vi "ReadLampState.vi"(8 "error in (no error)":errorcluster, 11 "RoomLight in":refnum<class "RoomLight.lvclass">) -> (0 "error out":errorcluster, 2 "LampState":bool, 3 "RoomLight out":refnum<class "RoomLight.lvclass">)   [LabVIEW 2013, in "RoomLight.lvclass"]
uses:
  RoomLight.lvclass
  RoomLight.lvclass/RoomLight.ctl
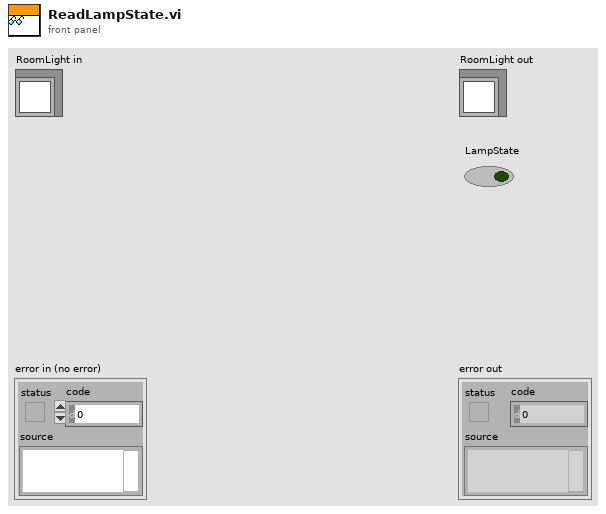
[diagram p1: front panel]
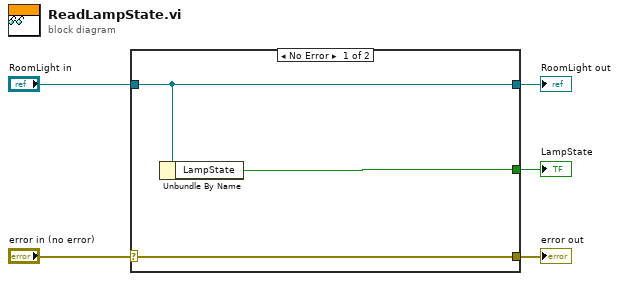
[diagram p0: block diagram]
diagram:
  n1 = case shown="No Error" "error in (no error)" {
    selector: "error in (no error)" -> [w8 w9]
    tunnel: [w8 w9] -> w4
    tunnel: [w7 w10] -> w2
    tunnel: "RoomLight in" -> [w7 w10]
    tunnel: [w6 _] -> w1
    frame No Error {
      n2 = Unbundle By Name(w7) -> ("LampState"=w6:bool)
    }
    frame Error {
    }
  }
  "error out" <- w4
  "RoomLight out" <- w2
  "LampState" <- w1
